vi "Time.Start End Order Check and Output Start End Date as Str.vi"(10 "End":timestamp, 11 "Start":timestamp) -> (2 "End Out":timestamp, 3 "Start Out":timestamp, 5 "Start_End Dates":string[](array[string]))   [LabVIEW 2019]
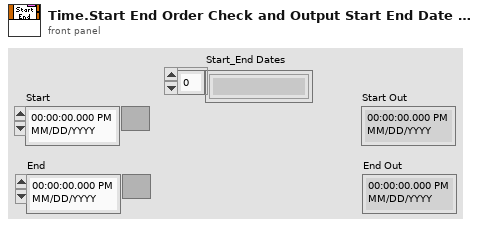
[diagram p1: front panel]
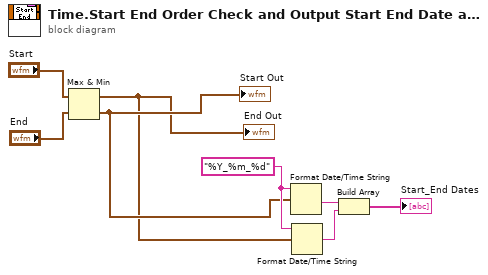
[diagram p0: block diagram]
diagram:
  w6 = "%Y_%m_%d" ("time format string (%c)")
  n1 = Max & Min(x="Start", y="End") -> (max(x,y)=w1:timestamp, min(x,y)=w2:timestamp)
  "Start Out" <- w2
  "End Out" <- w1
  n2 = Format Date/Time String(time format string (%c)=w6, seconds (now)=w2) -> (date/time string=w8:string)  [unwired: 1 in]
  n3 = Format Date/Time String(time format string (%c)=w6, seconds (now)=w1) -> (date/time string=w7:string)  [unwired: 1 in]
  n4 = Build Array(w8, w7) -> (→"Start_End Dates":string[])
